vi "Autonomous Independent.vi"() -> ()   [LabVIEW 2014]
doc: "This VI is called when autonomous begins, and will automatically be terminated when autonomous ends. You can carry out timed or sensor driven robot movement independently without needing to return to the caller."
uses:
  Public/Documents/FRC/Strict Typ Def Autonomous.ctl
  <vilib>/Rock Robotics/WPI/Joystick/WPI_JoystickGetSetRefNum.vi
  <vilib>/Rock Robotics/WPI/RobotDrive/WPI_RobotDriveArcadeDrive_Standard(NoSaturation).vi
panel:
  in  "Limit-Claw Closed":bool
  in  "Bottom Limit":bool
  in  "LImit-Claw Open":bool
  in  "Auto States":T1
  in  "Back Away at x time for y speed":bool
  in  "Start":bool
  out "Auto States 2":u16
  in  "PID Reached?":bool
  out "Current Movement, for debugging":T2 {"Y Joystick Value" scale=1.0..-1.0; "X Joystick Value" scale=-1.0..1.0}
  in  "Array of robot movements":T3(array[cluster]) {"Y Joystick Value" scale=1.0..-1.0; "X Joystick Value" scale=-1.0..1.0}
  # "Be sure to right-click and choose Data Operations>>Make Current Value default if you want to save the array values with the VI"
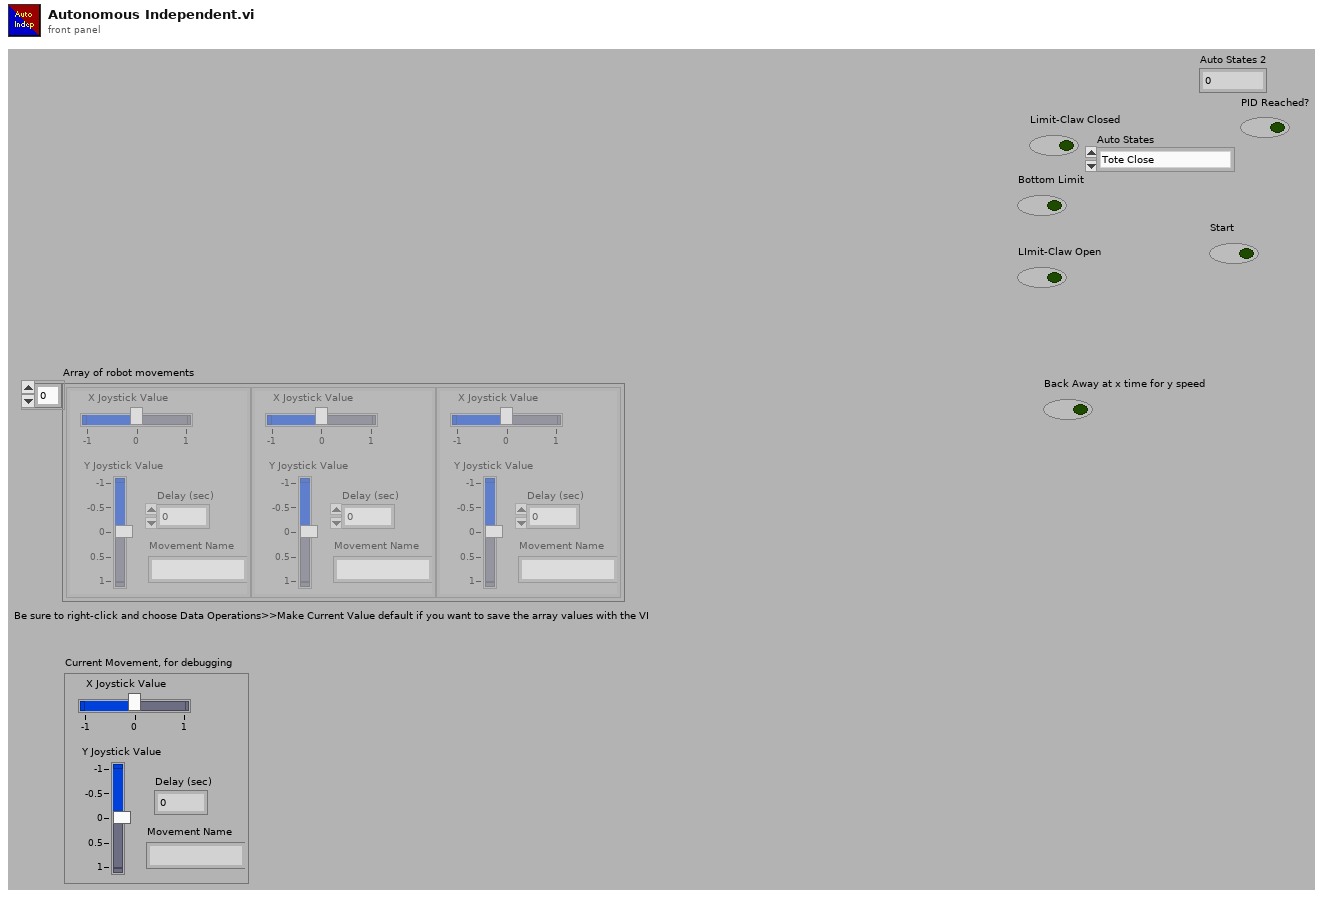
[diagram p1: front panel]
types:
  T1 = typedef "Strict Typ Def Autonomous.ctl" = enum16{"Tote Close", "Tote Raising", "Tote Turning", "Forward ", "Tote Lowering", "Tote Opening", "Tote Back Away", "Turn toward RC", "Forward to RC", "RC Close", "RC Raising", "RC Turning", "Forward with RC", "RC Lowering", "RC Opening", "RC Back Away", "Done", "Ready"}
  T2 = cluster{"X Joystick Value":dbl, "Y Joystick Value":dbl, "Delay (sec)":dbl, "Movement Name":string}
  T3 = cluster{"X Joystick Value":dbl, "Y Joystick Value":dbl, "Delay (sec)":dbl, "Movement Name":string}[]
  T4 = typedef "WPI_JoystickDevRef.ctl" = cluster{"Device":T5}
  T5 = typedef "WPI_JoystickDeviceEnum.ctl" = enum16{"USB 0", "USB 1", "USB 2", "USB 3", "USB 4", "USB 5"}
  T6 = typedef "WPI_RobotDriveDevRef.ctl" = cluster{"DevStatus":errorcluster, "Motors[]":T7[], "Square Inputs":bool, "Max Output":dbl}
  T7 = typedef "WPI_MotorControlDeviceRef.ctl" = cluster{"DeviceStatus":errorcluster, "Type":T8, "PWM":cluster{"Controller":T9, "PWM Channel":T10, "DeadBand":T11}, "CAN":cluster{"Device Number":u8, "Control Mode":T12, "Semaphore":T13, "Max Vout":dbl, "TalonSRX Control Mode":T14}, "Invert":bool, "TransformRef":T15, "InvTransformRef":T15}
  T8 = typedef "WPI_MotorControlType.ctl" = enum16{"PWM", "CAN", "CANTalonSRX"}
  T9 = typedef "FPGA_TypedefDigitalModule.ctl" = enum16{"Controller 1"}
  T10 = typedef "FPGA_DIOPWMChannel.ctl" = enum8{"PWM 0", "PWM 1", "PWM 2", "PWM 3", "PWM 4", "PWM 5", "PWM 6", "PWM 7", "PWM 8", "PWM 9", "PWM MXP 0", "PWM MXP 1", "PWM MXP 2", "PWM MXP 3", "PWM MXP 4", "PWM MXP 5", "PWM MXP 6", "PWM MXP 7", "PWM MXP 8", "PWM MXP 9", "Invalid"}
  T11 = typedef "WPI_PWMDeadband.ctl" = cluster{"Name":string, "maxPositivePwm":i32, "minPositivePwm":i32, "centerPwm":i32, "maxNegativePwm":i32, "minNegativePwm":i32, "angularRange":u16}
  T12 = typedef "WPI_CANJaguar_ControlMode.ctl" = enum8{"Percent VBus", "Current", "Speed", "Position", "Voltage"}
  T13 = typedef "Semaphore RefNum" = refnum<k1>
  T14 = typedef "WPI_CANTalonSRX_APIControlMode.ctl" = enum8{"Percent VBus", "Speed", "Position", "Slave", "Unchanged / Invalid"}
  T15 = typedef "WPI_PWMTransform_ConPane.ctl" = refnum<vi>
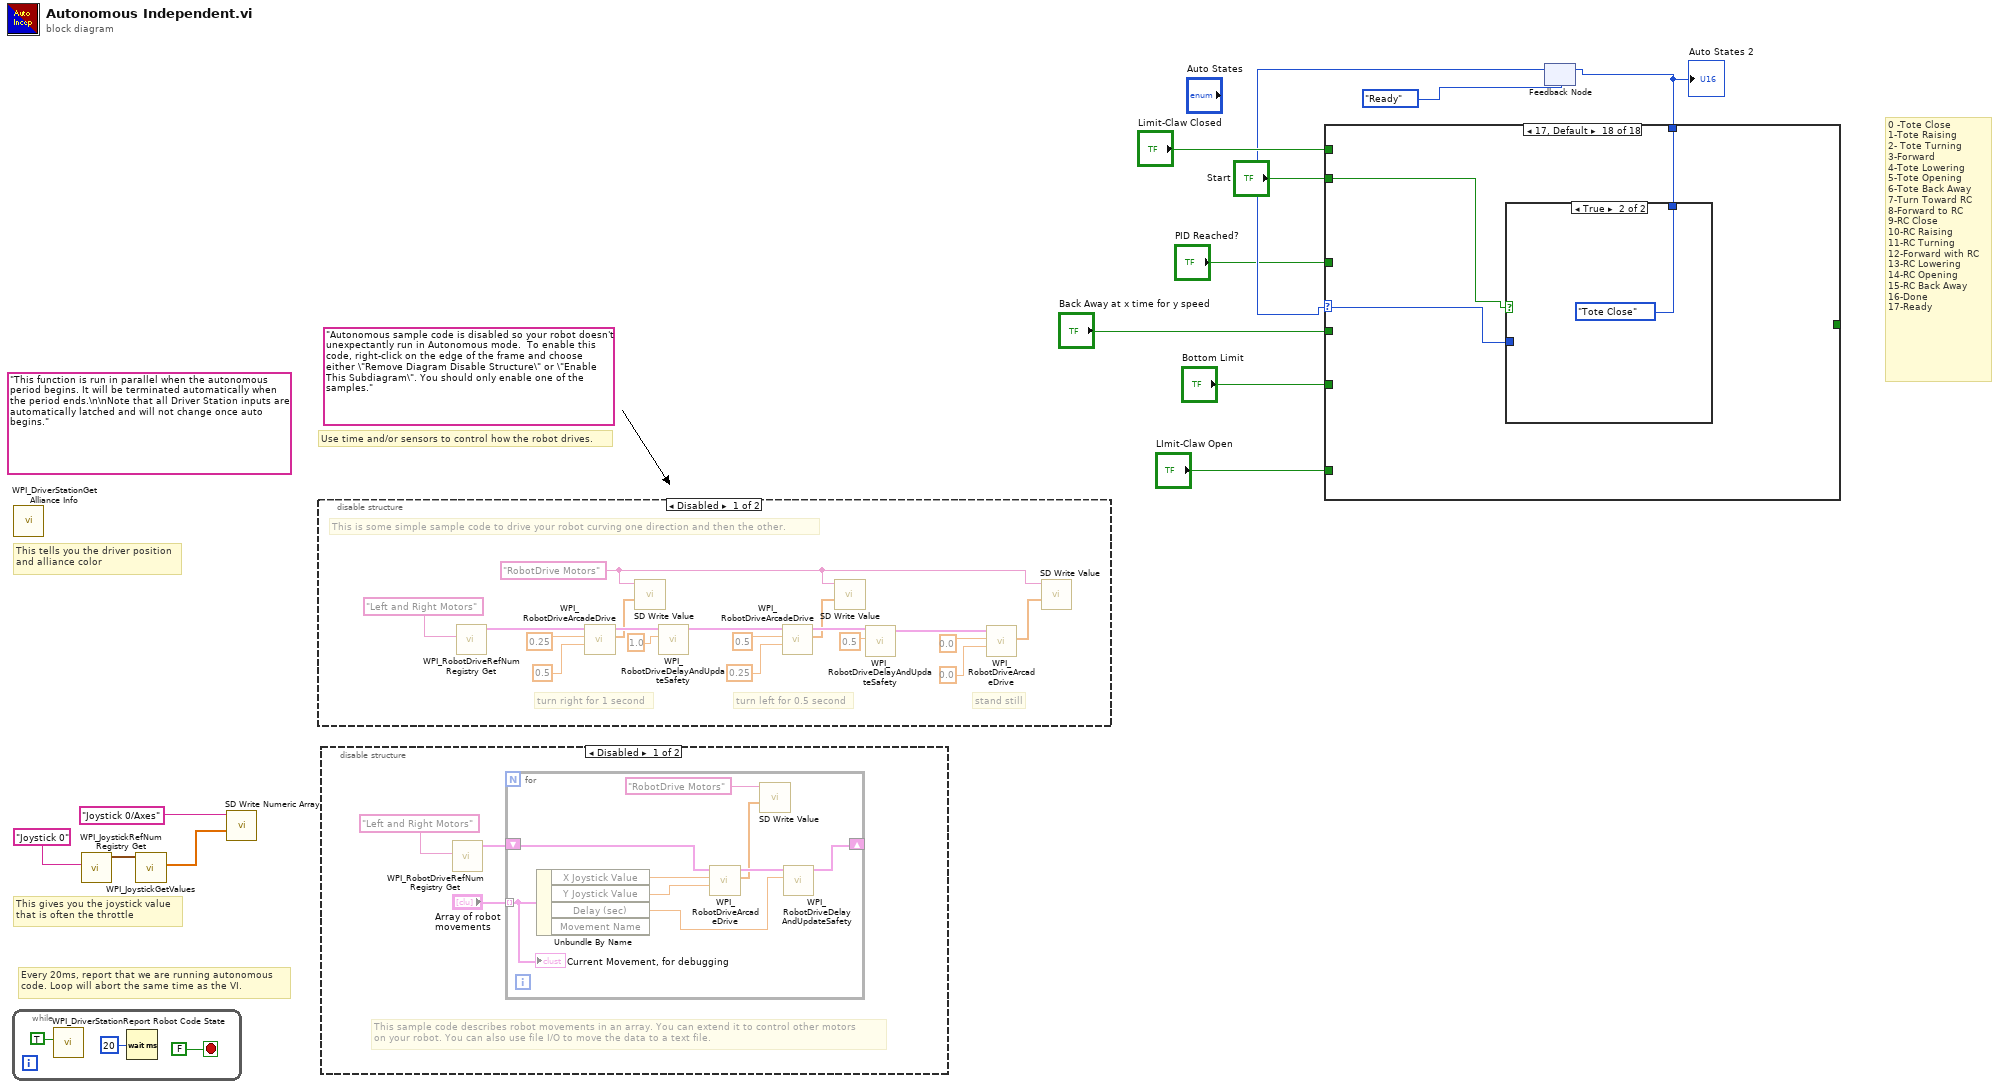
[diagram p0: block diagram]
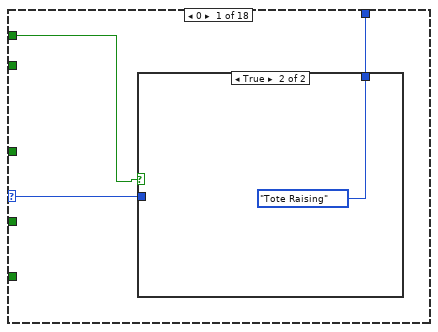
[diagram p2: hidden frame]
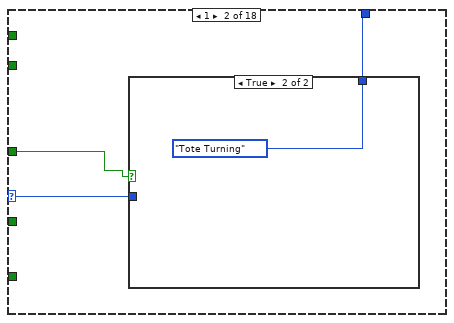
[diagram p4: hidden frame]
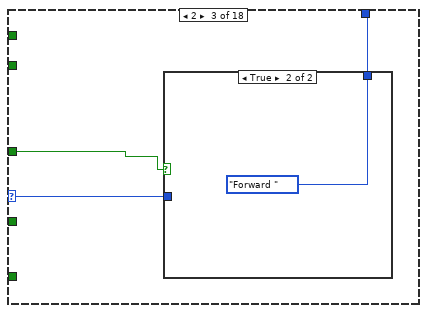
[diagram p6: hidden frame]
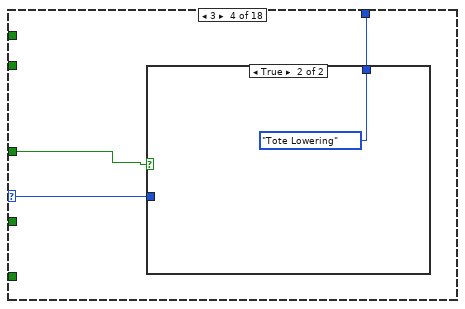
[diagram p8: hidden frame]
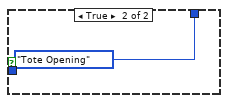
[diagram p11: hidden frame]
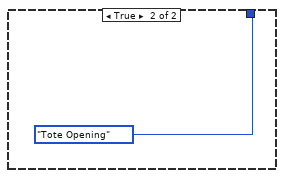
[diagram p12: hidden frame]
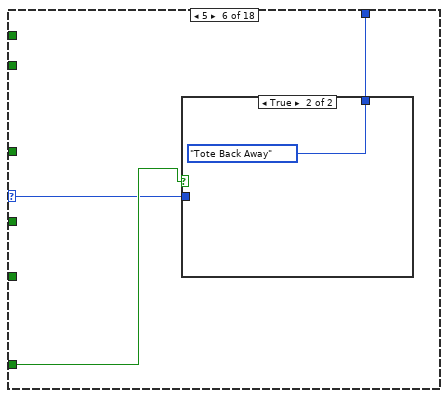
[diagram p13: hidden frame]
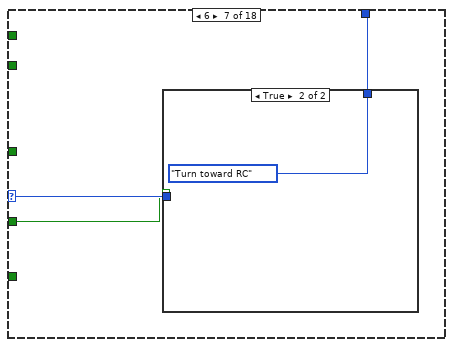
[diagram p15: hidden frame]
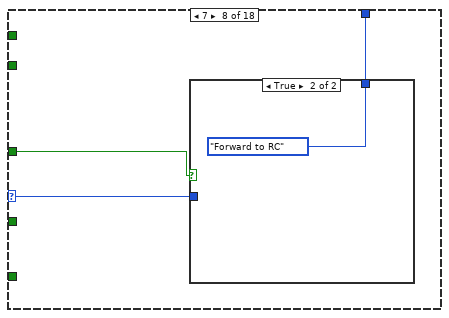
[diagram p17: hidden frame]
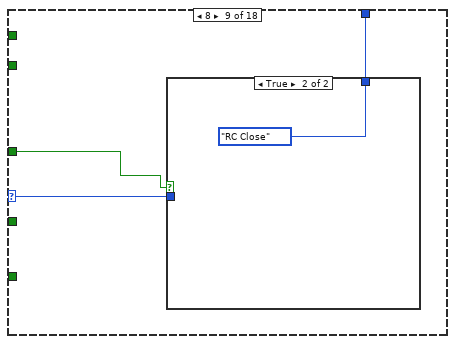
[diagram p19: hidden frame]
diagram:
  (unwired) "Autonomous sample code is disabled so your robot doesn't unexpectantly run in Autonomous mode.  To enable this code, right-click on the edge of the frame and choose either \"Remove Diagram Disable Structure\" or \"Enable This Subdiagram\". You should only enable one of the samples."
  (unwired) "This function is run in parallel when the autonomous period begins. It will be terminated automatically when the period ends.\n\nNote that all Driver Station inputs are automatically latched and will not change once auto begins."
  # "0 -Tote Close\n1-Tote Raising\n2- Tote Turning\n3-Forward\n4-Tote Lowering\n5-Tote Opening\n6-Tote Back Away\n7-Turn Toward RC\n8-Forward to RC\n9-RC Close\n10-RC Raising\n11-RC Turning\n12-Forward with RC\n13-RC Lowering\n14-RC Opening\n15-RC Back Away\n16-Done\n17-Ready"
  # "Every 20ms, report that we are running autonomous\ncode. Loop will abort the same time as the VI."
  # "This gives you the joystick value\nthat is often the throttle"
  # "Use time and/or sensors to control how the robot drives."
  # "This tells you the driver position\nand alliance color"
  n1 = while {
    stop <- FALSE stop-if-true
    n2 = call <vilib>:"WPI_DriverStationReport Robot Code State.vi"("Autonomous"=TRUE) -> ()  [unwired: 10 in, 1 out]
    n3 = Wait (ms)(milliseconds to wait=u32 20) -> ()  [unwired: 1 out]
  }
  n4 = call <vilib>:"WPI_DriverStationGet Alliance Info.vi"() -> ()  [unwired: 12 out]
  n5 = call <vilib>:"WPI_JoystickRefNum Registry Get.vi"("refnum name"="Joystick 0") -> ("JoystickDevRef"=w12:T4)  [unwired: 1 in, 9 out]
  n6 = call <vilib>:"WPI_JoystickGetValues.vi"("JoystickDevRef"=w12) -> ("Axes"=w10:dbl[])  [unwired: 6 in, 4 out]
  n7 = call <vilib>:"SD Write Numeric Array.vi"("Numeric Array"=w10, "Name"="Joystick 0/Axes") -> ()  [unwired: 8 in, 2 out]
  n8 = disable-structure shown="Disabled" {
    frame Disabled {
      w20 = "RobotDrive Motors" ("Name")
      # "This is some simple sample code to drive your robot curving one direction and then the other."
      # "stand still"
      # "turn left for 0.5 second"
      # "turn right for 1 second"
      n9 = call <vilib>:"WPI_RobotDriveRefNum Registry Get.vi"("refnum name"="Left and Right Motors") -> ("RobotDriveDevRef"=w21:T6)  [unwired: 1 in, 9 out]
      n10 = call-poly <vilib>:"WPI_RobotDriveArcadeDrive.vi"("Y axis value"=0.5 ("X axis value"), "X axis value"=0.25, "RobotDriveDevRef"=w21) -> ("Motor Values"=w19:dbl[], "RobotDriveDevRef"=w28:T6)  [unwired: 1 in, 6 out]
      n11 = call-poly <vilib>:"SD Write Value.vi"("Numeric Array"=w19, "Name"=w20) -> ()  [unwired: 8 in, 2 out]
      n12 = call <vilib>:"WPI_RobotDriveDelayAndUpdateSafety.vi"("Delay (s)"=1.0, "RobotDriveDevRef"=w28) -> ("RobotDriveDevRef 2"=w27:T6)  [unwired: 8 in, 1 out]
      n13 = call-poly <vilib>:"WPI_RobotDriveArcadeDrive.vi"("Y axis value"=0.25 ("X axis value"), "X axis value"=0.5, "RobotDriveDevRef"=w27) -> ("Motor Values"=w18:dbl[], "RobotDriveDevRef"=w26:T6)  [unwired: 1 in, 6 out]
      n14 = call-poly <vilib>:"SD Write Value.vi"("Numeric Array"=w18, "Name"=w20) -> ()  [unwired: 8 in, 2 out]
      n15 = call <vilib>:"WPI_RobotDriveDelayAndUpdateSafety.vi"("Delay (s)"=0.5, "RobotDriveDevRef"=w26) -> ("RobotDriveDevRef 2"=w25:T6)  [unwired: 8 in, 1 out]
      n16 = call-poly <vilib>:"WPI_RobotDriveArcadeDrive.vi"("Y axis value"=0.0 ("X axis value"), "X axis value"=0.0, "RobotDriveDevRef"=w25) -> ("Motor Values"=w17:dbl[])  [unwired: 1 in, 7 out]
      n17 = call-poly <vilib>:"SD Write Value.vi"("Numeric Array"=w17, "Name"=w20) -> ()  [unwired: 8 in, 2 out]
    }
    frame Enabled {
    }
  }
  n18 = disable-structure shown="Disabled" {
    frame Disabled {
      # "This sample code describes robot movements in an array. You can extend it to control other motors\non your robot. You can also use file I/O to move the data to a text file."
      n19 = call <vilib>:"WPI_RobotDriveRefNum Registry Get.vi"("refnum name"="Left and Right Motors") -> ("RobotDriveDevRef"=w36:T6)  [unwired: 1 in, 9 out]
      n20 = for {
        shift-right: [w43] -> _
        shift-left: w36 -> [w44]
        tunnel: "Array of robot movements" -> [w39] mode=indexing
        n21 = Unbundle By Name(w39) -> ("X Joystick Value"=w42:dbl, "Y Joystick Value"=w41:dbl, "Delay (sec)"=w40:dbl)  [unwired: 1 out]
        n22 = call-poly <vilib>:"WPI_RobotDriveArcadeDrive.vi"("Y axis value"=w41, "X axis value"=w42, "RobotDriveDevRef"=w44) -> ("Motor Values"=w38:dbl[], "RobotDriveDevRef"=w45:T6)  [unwired: 1 in, 6 out]
        n23 = call-poly <vilib>:"SD Write Value.vi"("Numeric Array"=w38, "Name"="RobotDrive Motors") -> ()  [unwired: 8 in, 2 out]
        n24 = call <vilib>:"WPI_RobotDriveDelayAndUpdateSafety.vi"("Delay (s)"=w40, "RobotDriveDevRef"=w45) -> ("RobotDriveDevRef 2"=w43:T6)  [unwired: 8 in, 1 out]
        "Current Movement, for debugging" <- w39
      }
    }
    frame Enabled {
    }
  }
  n25 = feedback #1(Strict_Typ_Def_Autonomous."Ready" ("Auto States")) -> (w5:u16)
  n26 = case shown="17, Default" w5 {
    selector: w5 -> [w47 w53 w58 w63 w68 w77 w83 w88 w93 w97 w103 w108 w113 w119 w127 w133 w137 w140]
    tunnel: "Limit-Claw Closed" -> [w49 _ _ _ _ _ _ _ _ w99 _ _ _ _ _ _ _ _]
    tunnel: "Bottom Limit" -> [_ _ _ _ w70 _ _ _ _ _ _ _ _ w120 _ _ _ _]
    tunnel: "LImit-Claw Open" -> [_ _ _ _ _ w79 _ _ _ _ _ _ _ _ w129 _ _ _]
    tunnel: [_ _ _ _ _ _ _ _ _ _ _ _ _ _ _ _ TRUE _] -> _
    tunnel: [w48 w54 w59 w64 w69 w78 w84 w89 w94 w98 w104 w109 w114 w118 w128 w134 w137 w141] -> w6
    tunnel: "Back Away at x time for y speed" -> [_ _ _ _ _ _ w82 _ _ _ _ _ _ _ _ w132 _ _]
    tunnel: "Start" -> [_ _ _ _ _ _ _ _ _ _ _ _ _ _ _ _ _ w139]
    tunnel: "PID Reached?" -> [_ w52 w57 w62 w67 _ _ w87 w92 _ w102 w107 w112 w117 _ _ _ _]
    frame 0 {
      n27 = case shown="True" w49 {
        tunnel: [w50 Strict_Typ_Def_Autonomous."Tote Raising" ("Auto States")] -> w48
        tunnel: w47 -> [w50 _]
        frame False {
        }
        frame True {
        }
      }
    }
    frame 1 {
      n28 = case shown="True" w52 {
        tunnel: [w55 Strict_Typ_Def_Autonomous."Tote Turning" ("Auto States")] -> w54
        tunnel: w53 -> [w55 _]
        frame False {
        }
        frame True {
        }
      }
    }
    frame 2 {
      n29 = case shown="True" w57 {
        tunnel: [w60 Strict_Typ_Def_Autonomous."Forward " ("Auto States")] -> w59
        tunnel: w58 -> [w60 _]
        frame False {
        }
        frame True {
        }
      }
    }
    frame 3 {
      n30 = case shown="True" w62 {
        tunnel: [w65 Strict_Typ_Def_Autonomous."Tote Lowering" ("Auto States")] -> w64
        tunnel: w63 -> [w65 _]
        frame False {
        }
        frame True {
        }
      }
    }
    frame 4 {
      n31 = case shown="False" w70 {
        tunnel: [w73 Strict_Typ_Def_Autonomous."Tote Opening" ("Auto States")] -> w69
        tunnel: w68 -> [w72 _]
        tunnel: w67 -> [w71 _]
        frame False {
          n32 = case shown="False" w71 {
            tunnel: [w74 Strict_Typ_Def_Autonomous."Tote Opening" ("Auto States")] -> w73
            tunnel: w72 -> [w74 _]
            frame False {
            }
            frame True {
            }
          }
        }
        frame True {
        }
      }
    }
    frame 5 {
      n33 = case shown="True" w79 {
        tunnel: [w80 Strict_Typ_Def_Autonomous."Tote Back Away" ("Auto States")] -> w78
        tunnel: w77 -> [w80 _]
        frame False {
        }
        frame True {
        }
      }
    }
    frame 6 {
      n34 = case shown="True" w82 {
        tunnel: [w85 Strict_Typ_Def_Autonomous."Turn toward RC" ("Auto States")] -> w84
        tunnel: w83 -> [w85 _]
        frame False {
        }
        frame True {
        }
      }
    }
    frame 7 {
      n35 = case shown="True" w87 {
        tunnel: [w90 Strict_Typ_Def_Autonomous."Forward to RC" ("Auto States")] -> w89
        tunnel: w88 -> [w90 _]
        frame False {
        }
        frame True {
        }
      }
    }
    frame 8 {
      n36 = case shown="True" w92 {
        tunnel: [w95 Strict_Typ_Def_Autonomous."RC Close" ("Auto States")] -> w94
        tunnel: w93 -> [w95 _]
        frame False {
        }
        frame True {
        }
      }
    }
    frame 9 {
      n37 = case shown="False" w99 {
        tunnel: [w100 Strict_Typ_Def_Autonomous."RC Raising" ("Auto States")] -> w98
        tunnel: w97 -> [w100 _]
        frame False {
        }
        frame True {
        }
      }
    }
    frame 10 {
      # "Do we want Limit High?"
      n38 = case shown="True" w102 {
        tunnel: [w105 Strict_Typ_Def_Autonomous."RC Turning" ("Auto States")] -> w104
        tunnel: w103 -> [w105 _]
        frame False {
        }
        frame True {
        }
      }
    }
    frame 11 {
      n39 = case shown="True" w107 {
        tunnel: [w110 Strict_Typ_Def_Autonomous."Forward with RC" ("Auto States")] -> w109
        tunnel: w108 -> [w110 _]
        frame False {
        }
        frame True {
        }
      }
    }
    frame 12 {
      n40 = case shown="True" w112 {
        tunnel: [w115 Strict_Typ_Def_Autonomous."RC Lowering" ("Auto States")] -> w114
        tunnel: w113 -> [w115 _]
        frame False {
        }
        frame True {
        }
      }
    }
    frame 13 {
      n41 = case shown="False" w120 {
        tunnel: w119 -> [w122 _]
        tunnel: [w123 Strict_Typ_Def_Autonomous."RC Opening" ("Auto States")] -> w118
        tunnel: w117 -> [w121 _]
        frame False {
          n42 = case shown="False" w121 {
            tunnel: [w124 Strict_Typ_Def_Autonomous."RC Opening" ("Auto States")] -> w123
            tunnel: w122 -> [w124 _]
            frame False {
            }
            frame True {
            }
          }
        }
        frame True {
        }
      }
    }
    frame 14 {
      n43 = case shown="False" w129 {
        tunnel: [w130 Strict_Typ_Def_Autonomous."RC Back Away" ("Auto States")] -> w128
        tunnel: w127 -> [w130 _]
        frame False {
        }
        frame True {
        }
      }
    }
    frame 15 {
      n44 = case shown="True" w132 {
        tunnel: [w135 Strict_Typ_Def_Autonomous."Done" ("Auto States")] -> w134
        tunnel: w133 -> [w135 _]
        frame False {
        }
        frame True {
        }
      }
    }
    frame 16 {
    }
    frame 17, Default {
      n45 = case shown="True" w139 {
        tunnel: [w142 Strict_Typ_Def_Autonomous."Tote Close" ("Auto States")] -> w141
        tunnel: w140 -> [w142 _]
        frame False {
        }
        frame True {
        }
      }
    }
  }
  "Auto States 2" <- w6
  n46 = feedback-in #1(w6) -> ()
